vi "click_button_coordinates.vi"(8 "error in (no error)":errorcluster, 11 "Boolean in":refnum<vi>) -> (0 "error out":errorcluster, 2 "Vertical":dbl, 3 "Horizontal":dbl)   [LabVIEW 2020, in "ui-testing.lvlib"]
uses:
  ui-testing.lvlib
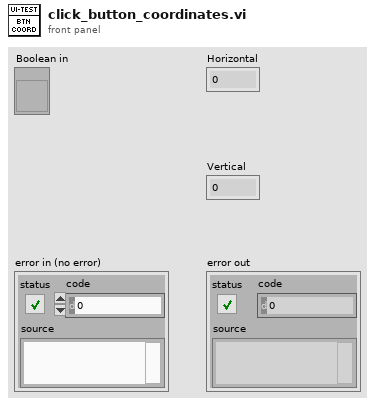
[diagram p1: front panel]
types:
  T1 = typedef "LVRectTypeDef.ctl" = cluster{"Left":i16, "Top":i16, "Right":i16, "Bottom":i16}
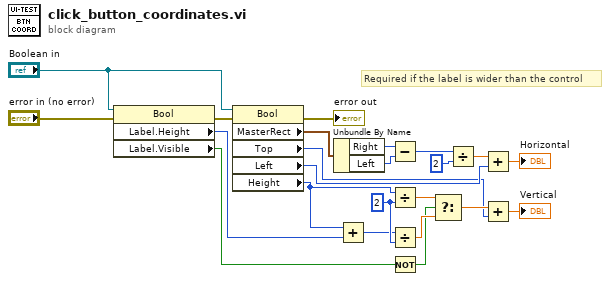
[diagram p0: block diagram]
diagram:
  w16 = u32 2 ("y")
  # "Required if the label is wider than the control"
  n1 = property class="Bool"(reference="Boolean in", error in="error in (no error)") -> (error out=w8:errorcluster, "Label.Height"=w14:u32, "Label.Visible"=w11:bool)  [unwired: 1 out]
  n2 = property on="Property Node" class="Bool"(reference="Boolean in", error in=w8) -> (error out=→"error out":errorcluster, "MasterRect"=w23:T1, "Top"=w1:i32, "Left"=w5:i32, "Height"=w13:u32)  [unwired: 1 out]
  n3 = Unbundle By Name(w23) -> ("Right"=w19:i16, "Left"=w20:i16)
  n4 = Add(x=w13, y=w14) -> (x+y=w15:u32)
  n5 = Subtract(x=w19, y=w20) -> (x-y=w21:i16)
  n6 = Divide(x=w13, y=w16) -> (x/y=w10:dbl)
  n7 = Divide(x=w15, y=w16) -> (x/y=w17:dbl)
  n8 = Not(x=w11) -> (.not. x?=w12:bool)
  n9 = Select(t=w10, s=w12, f=w17) -> (s? t:f=w18:dbl)
  n10 = Divide(x=w21, y=i16 2) -> (x/y=w4:dbl)
  n11 = Add(x=w4, y=w5) -> (x+y=→"Horizontal":dbl)
  n12 = Add(x=w18, y=w1) -> (x+y=→"Vertical":dbl)
